vi "Three part.vi"() -> ()   [LabVIEW 2009]
uses:
  <vilib>/vision/Image Controls.llb/IMAQ Image.ctl
  <vilib>/Instr/_visa.llb/VISA Configure Serial Port (Instr).vi
  <vilib>/Analysis/3filter.llb/Filter Passband Type.ctl
  <vilib>/Analysis/3filter.llb/Butterworth Filter (DBL).vi
  <vilib>/vision/NI_Vision_Development_Module.lvlib
  <vilib>/Analysis/NI_AALBase.lvlib
panel:
  in  "Orange Guitar":T1={"Global Rectangle"=[587, 282, 628, 378], "Contours"=[{"ID"=enum."External", "Type"=2, "Coordinates"=[627, 377, 587, 282]}]} {"Contours"."Type" items=["No Selection", "Point", "Line", "Rectangle", "Oval", "Polygon", "Freehand Region", "Annulus", "Unused2", "Unused3", "Broken Line", "Freehand Line", "Rotated Rectangle"]}
  in  "Yellow Guitar":T1={"Global Rectangle"=[546, 282, 563, 376], "Contours"=[{"ID"=enum."External", "Type"=2, "Coordinates"=[562, 375, 546, 282]}]} {"Contours"."Type" items=["No Selection", "Point", "Line", "Rectangle", "Oval", "Polygon", "Freehand Region", "Annulus", "Unused2", "Unused3", "Broken Line", "Freehand Line", "Rotated Rectangle"]}
  in  "Green Guitar":T1={"Global Rectangle"=[498, 284, 505, 376], "Contours"=[{"ID"=enum."External", "Type"=2, "Coordinates"=[498, 375, 504, 284]}]} {"Contours"."Type" items=["No Selection", "Point", "Line", "Rectangle", "Oval", "Polygon", "Freehand Region", "Annulus", "Unused2", "Unused3", "Broken Line", "Freehand Line", "Rotated Rectangle"]}
  in  "Blue Guitar":T1={"Global Rectangle"=[569, 290, 594, 372], "Contours"=[{"ID"=enum."External", "Type"=2, "Coordinates"=[593, 371, 569, 290]}]} {"Contours"."Type" items=["No Selection", "Point", "Line", "Rectangle", "Oval", "Polygon", "Freehand Region", "Annulus", "Unused2", "Unused3", "Broken Line", "Freehand Line", "Rotated Rectangle"]}
  in  "Red Guitar":T1={"Global Rectangle"=[526, 284, 530, 370], "Contours"=[{"ID"=enum."External", "Type"=2, "Coordinates"=[529, 369, 526, 284]}]} {"Contours"."Type" items=["No Selection", "Point", "Line", "Rectangle", "Oval", "Polygon", "Freehand Region", "Annulus", "Unused2", "Unused3", "Broken Line", "Freehand Line", "Rotated Rectangle"]}
  in  "sampling  9":dbl=1.0 format="%0.2f"
  in  "high 14":dbl=60.0 format="%0.2f"
  out "Blue Guitar":dbl[](graph)
  in  "low 3":dbl=0.12500000000000006 format="%0.4f"
  out "Yellow Guitar":dbl[](graph)
  out "Yellow Guitar LED":bool
  in  "sampling 12":dbl=1.0 format="%0.2f"
  in  "high 13":dbl=60.0 format="%0.2f"
  in  "low  12":dbl=0.12500000000000006 format="%0.4f"
  out "Yellow Guitar":T1={"Global Rectangle"=[243, 262, 261, 384], "Contours"=[{"ID"=enum."External", "Type"=2, "Coordinates"=[260, 383, 243, 262]}]} {"Contours"."Type" items=["No Selection", "Point", "Line", "Rectangle", "Oval", "Polygon", "Freehand Region", "Annulus", "Unused2", "Unused3", "Broken Line", "Freehand Line", "Rotated Rectangle"]}
  out "Blue Guitar":T1={"Global Rectangle"=[168, 264, 180, 378], "Contours"=[{"ID"=enum."External", "Type"=2, "Coordinates"=[168, 377, 179, 264]}]} {"Contours"."Type" items=["No Selection", "Point", "Line", "Rectangle", "Oval", "Polygon", "Freehand Region", "Annulus", "Unused2", "Unused3", "Broken Line", "Freehand Line", "Rotated Rectangle"]}
  out "Green Guitar":dbl[](graph)
  out "Green Guitar LED":bool
  in  "sampling 11":dbl=1.0 format="%0.2f"
  in  "high 12":dbl=60.0 format="%0.2f"
  in  "low  11":dbl=0.12500000000000006 format="%0.4f"
  out "Green Guitar":T1={"Global Rectangle"=[406, 309, 423, 383], "Contours"=[{"ID"=enum."External", "Type"=2, "Coordinates"=[422, 382, 406, 309]}]} {"Contours"."Type" items=["No Selection", "Point", "Line", "Rectangle", "Oval", "Polygon", "Freehand Region", "Annulus", "Unused2", "Unused3", "Broken Line", "Freehand Line", "Rotated Rectangle"]}
  out "Red Guitar":dbl[](graph)
  out "Red Guitar LED":bool
  in  "sampling 10":dbl=1.0 format="%0.2f"
  in  "high 11":dbl=60.0 format="%0.2f"
  in  "low  10":dbl=0.12500000000000006 format="%0.4f"
  out "Red Guitar":T1={"Global Rectangle"=[300, 297, 320, 380], "Contours"=[{"ID"=enum."External", "Type"=2, "Coordinates"=[300, 379, 319, 297]}]} {"Contours"."Type" items=["No Selection", "Point", "Line", "Rectangle", "Oval", "Polygon", "Freehand Region", "Annulus", "Unused2", "Unused3", "Broken Line", "Freehand Line", "Rotated Rectangle"]}
  out "Blue Guitar LED":bool
  out "Orange Guitar":dbl[](graph)
  out "Orange Guitar LED":bool
  in  "sampling 9":dbl=1.0 format="%0.2f"
  in  "high 10":dbl=60.0 format="%0.2f"
  in  "low  9":dbl=0.12500000000000006 format="%0.4f"
  out "Orange Guitar":T1={"Global Rectangle"=[300, 297, 320, 380], "Contours"=[{"ID"=enum."External", "Type"=2, "Coordinates"=[300, 379, 319, 297]}]} {"Contours"."Type" items=["No Selection", "Point", "Line", "Rectangle", "Oval", "Polygon", "Freehand Region", "Annulus", "Unused2", "Unused3", "Broken Line", "Freehand Line", "Rotated Rectangle"]}
  in  "Orange Bass":T1={"Global Rectangle"=[220, 296, 225, 371], "Contours"=[{"ID"=enum."External", "Type"=2, "Coordinates"=[224, 370, 220, 296]}]} {"Contours"."Type" items=["No Selection", "Point", "Line", "Rectangle", "Oval", "Polygon", "Freehand Region", "Annulus", "Unused2", "Unused3", "Broken Line", "Freehand Line", "Rotated Rectangle"]}
  out "Orange Bass":dbl[](graph)
  out "Orange Bass LED":bool
  in  "sampling 8":dbl=1.0 format="%0.2f"
  in  "high 9":dbl=60.0 format="%0.2f"
  in  "low  8":dbl=0.12500000000000006 format="%0.4f"
  out "Orange Bass":T1={"Global Rectangle"=[300, 297, 320, 380], "Contours"=[{"ID"=enum."External", "Type"=2, "Coordinates"=[300, 379, 319, 297]}]} {"Contours"."Type" items=["No Selection", "Point", "Line", "Rectangle", "Oval", "Polygon", "Freehand Region", "Annulus", "Unused2", "Unused3", "Broken Line", "Freehand Line", "Rotated Rectangle"]}
  in  "Green Bass":T1={"Global Rectangle"=[100, 292, 131, 371], "Contours"=[{"ID"=enum."External", "Type"=2, "Coordinates"=[100, 370, 130, 292]}]} {"Contours"."Type" items=["No Selection", "Point", "Line", "Rectangle", "Oval", "Polygon", "Freehand Region", "Annulus", "Unused2", "Unused3", "Broken Line", "Freehand Line", "Rotated Rectangle"]}
  in  "Blue Bass":T1={"Global Rectangle"=[193, 293, 199, 374], "Contours"=[{"ID"=enum."External", "Type"=2, "Coordinates"=[193, 373, 198, 293]}]} {"Contours"."Type" items=["No Selection", "Point", "Line", "Rectangle", "Oval", "Polygon", "Freehand Region", "Annulus", "Unused2", "Unused3", "Broken Line", "Freehand Line", "Rotated Rectangle"]}
  in  "Red Bass":T1={"Global Rectangle"=[129, 294, 154, 376], "Contours"=[{"ID"=enum."External", "Type"=2, "Coordinates"=[129, 375, 153, 294]}]} {"Contours"."Type" items=["No Selection", "Point", "Line", "Rectangle", "Oval", "Polygon", "Freehand Region", "Annulus", "Unused2", "Unused3", "Broken Line", "Freehand Line", "Rotated Rectangle"]}
  in  "Yellow Bass":T1={"Global Rectangle"=[160, 295, 175, 378], "Contours"=[{"ID"=enum."External", "Type"=2, "Coordinates"=[160, 377, 174, 295]}]} {"Contours"."Type" items=["No Selection", "Point", "Line", "Rectangle", "Oval", "Polygon", "Freehand Region", "Annulus", "Unused2", "Unused3", "Broken Line", "Freehand Line", "Rotated Rectangle"]}
  in  "sampling  8":dbl=1.0 format="%0.2f"
  in  "high 8":dbl=60.0 format="%0.2f"
  out "Blue Bass":dbl[](graph)
  in  "low 2":dbl=0.12500000000000006 format="%0.4f"
  out "Yellow Bass":dbl[](graph)
  out "Yellow Bass LED":bool
  in  "sampling 7":dbl=1.0 format="%0.2f"
  in  "high 7":dbl=60.0 format="%0.2f"
  in  "low  7":dbl=0.12500000000000006 format="%0.4f"
  out "Yellow Bass":T1={"Global Rectangle"=[243, 262, 261, 384], "Contours"=[{"ID"=enum."External", "Type"=2, "Coordinates"=[260, 383, 243, 262]}]} {"Contours"."Type" items=["No Selection", "Point", "Line", "Rectangle", "Oval", "Polygon", "Freehand Region", "Annulus", "Unused2", "Unused3", "Broken Line", "Freehand Line", "Rotated Rectangle"]}
  out "Blue Bass":T1={"Global Rectangle"=[168, 264, 180, 378], "Contours"=[{"ID"=enum."External", "Type"=2, "Coordinates"=[168, 377, 179, 264]}]} {"Contours"."Type" items=["No Selection", "Point", "Line", "Rectangle", "Oval", "Polygon", "Freehand Region", "Annulus", "Unused2", "Unused3", "Broken Line", "Freehand Line", "Rotated Rectangle"]}
  out "Green Bass":dbl[](graph)
  out "Green Bass LED":bool
  in  "sampling 6":dbl=1.0 format="%0.2f"
  in  "high 6":dbl=60.0 format="%0.2f"
  in  "low  6":dbl=0.12500000000000006 format="%0.4f"
  out "Green Bass":T1={"Global Rectangle"=[406, 309, 423, 383], "Contours"=[{"ID"=enum."External", "Type"=2, "Coordinates"=[422, 382, 406, 309]}]} {"Contours"."Type" items=["No Selection", "Point", "Line", "Rectangle", "Oval", "Polygon", "Freehand Region", "Annulus", "Unused2", "Unused3", "Broken Line", "Freehand Line", "Rotated Rectangle"]}
  out "Red Bass":dbl[](graph)
  out "Red Bass LED":bool
  in  "sampling 5":dbl=1.0 format="%0.2f"
  in  "high 5":dbl=60.0 format="%0.2f"
  in  "low  5":dbl=0.12500000000000006 format="%0.4f"
  out "Red Bass":T1={"Global Rectangle"=[300, 297, 320, 380], "Contours"=[{"ID"=enum."External", "Type"=2, "Coordinates"=[300, 379, 319, 297]}]} {"Contours"."Type" items=["No Selection", "Point", "Line", "Rectangle", "Oval", "Polygon", "Freehand Region", "Annulus", "Unused2", "Unused3", "Broken Line", "Freehand Line", "Rotated Rectangle"]}
  out "Blue Bass LED":bool
  in  "Mask":T1 {"Contours"."Type" items=["No Selection", "Point", "Line", "Rectangle", "Oval", "Polygon", "Freehand Region", "Annulus", "Unused2", "Unused3", "Broken Line", "Freehand Line", "Rotated Rectangle"]}
  out "Image 2":T2(plugin-control)
  out "Red Line":T1={"Global Rectangle"=[300, 297, 320, 380], "Contours"=[{"ID"=enum."External", "Type"=2, "Coordinates"=[300, 379, 319, 297]}]} {"Contours"."Type" items=["No Selection", "Point", "Line", "Rectangle", "Oval", "Polygon", "Freehand Region", "Annulus", "Unused2", "Unused3", "Broken Line", "Freehand Line", "Rotated Rectangle"]}
  in  "Red Line":T1={"Global Rectangle"=[300, 297, 320, 380], "Contours"=[{"ID"=enum."External", "Type"=2, "Coordinates"=[300, 379, 319, 297]}]} {"Contours"."Type" items=["No Selection", "Point", "Line", "Rectangle", "Oval", "Polygon", "Freehand Region", "Annulus", "Unused2", "Unused3", "Broken Line", "Freehand Line", "Rotated Rectangle"]}
  out "Waveform Red":dbl[](graph)
  out "LED Red":bool
  in  "sampling 4":dbl=1.0 format="%0.2f"
  in  "high 4":dbl=60.0 format="%0.2f"
  in  "low  4":dbl=0.12500000000000006 format="%0.4f"
  out "Green Line":T1={"Global Rectangle"=[406, 309, 423, 383], "Contours"=[{"ID"=enum."External", "Type"=2, "Coordinates"=[422, 382, 406, 309]}]} {"Contours"."Type" items=["No Selection", "Point", "Line", "Rectangle", "Oval", "Polygon", "Freehand Region", "Annulus", "Unused2", "Unused3", "Broken Line", "Freehand Line", "Rotated Rectangle"]}
  in  "Blue Line":T1={"Global Rectangle"=[374, 278, 383, 377], "Contours"=[{"ID"=enum."External", "Type"=2, "Coordinates"=[382, 376, 374, 278]}]} {"Contours"."Type" items=["No Selection", "Point", "Line", "Rectangle", "Oval", "Polygon", "Freehand Region", "Annulus", "Unused2", "Unused3", "Broken Line", "Freehand Line", "Rotated Rectangle"]}
  in  "Green Line":T1={"Global Rectangle"=[406, 309, 423, 383], "Contours"=[{"ID"=enum."External", "Type"=2, "Coordinates"=[422, 382, 406, 309]}]} {"Contours"."Type" items=["No Selection", "Point", "Line", "Rectangle", "Oval", "Polygon", "Freehand Region", "Annulus", "Unused2", "Unused3", "Broken Line", "Freehand Line", "Rotated Rectangle"]}
  in  "low  3":dbl=0.12500000000000006 format="%0.4f"
  out "Waveform Green":dbl[](graph)
  out "LED Green":bool
  in  "sampling 3":dbl=1.0 format="%0.2f"
  in  "high 3":dbl=60.0 format="%0.2f"
  in  "Yellow Line":T1={"Global Rectangle"=[342, 292, 349, 377], "Contours"=[{"ID"=enum."External", "Type"=2, "Coordinates"=[342, 376, 348, 292]}]} {"Contours"."Type" items=["No Selection", "Point", "Line", "Rectangle", "Oval", "Polygon", "Freehand Region", "Annulus", "Unused2", "Unused3", "Broken Line", "Freehand Line", "Rotated Rectangle"]}
  out "Blue Line":T1={"Global Rectangle"=[168, 264, 180, 378], "Contours"=[{"ID"=enum."External", "Type"=2, "Coordinates"=[168, 377, 179, 264]}]} {"Contours"."Type" items=["No Selection", "Point", "Line", "Rectangle", "Oval", "Polygon", "Freehand Region", "Annulus", "Unused2", "Unused3", "Broken Line", "Freehand Line", "Rotated Rectangle"]}
  out "cluster":T3
  in  "baud rate (9600)":u32=9600
  in  "VISA resource name":refnum<visa-resource-name>
  out "number":u32
  out "decimal integer string":string
  out "Image Dst Out":T2
  out "Yellow Line":T1={"Global Rectangle"=[243, 262, 261, 384], "Contours"=[{"ID"=enum."External", "Type"=2, "Coordinates"=[260, 383, 243, 262]}]} {"Contours"."Type" items=["No Selection", "Point", "Line", "Rectangle", "Oval", "Polygon", "Freehand Region", "Annulus", "Unused2", "Unused3", "Broken Line", "Freehand Line", "Rotated Rectangle"]}
  in  "low  2":dbl=0.12500000000000006 format="%0.4f"
  in  "high 2":dbl=60.0 format="%0.2f"
  in  "sampling 2":dbl=1.0 format="%0.2f"
  out "LED Yellow":bool
  out "Waveform Yellow":dbl[](graph)
  in  "playtime":dbl=30.0
  out "Frame Number":i32
  in  "Frame Start":i32=2400
  out "Blue Drum":bool
  in  "low":dbl=0.12500000000000006 format="%0.4f"
  out "Blue Drum":dbl[](graph)
  in  "high":dbl=60.0 format="%0.2f"
  in  "sampling":dbl=1.0 format="%0.2f"
  in  "stop":bool
  in  "AVI Path":path
  # "BLUE"
  # "YELLOW"
  # "GREEN"
  # "RED"
  # "Drums"
  # "Bass"
  # "Guitar"
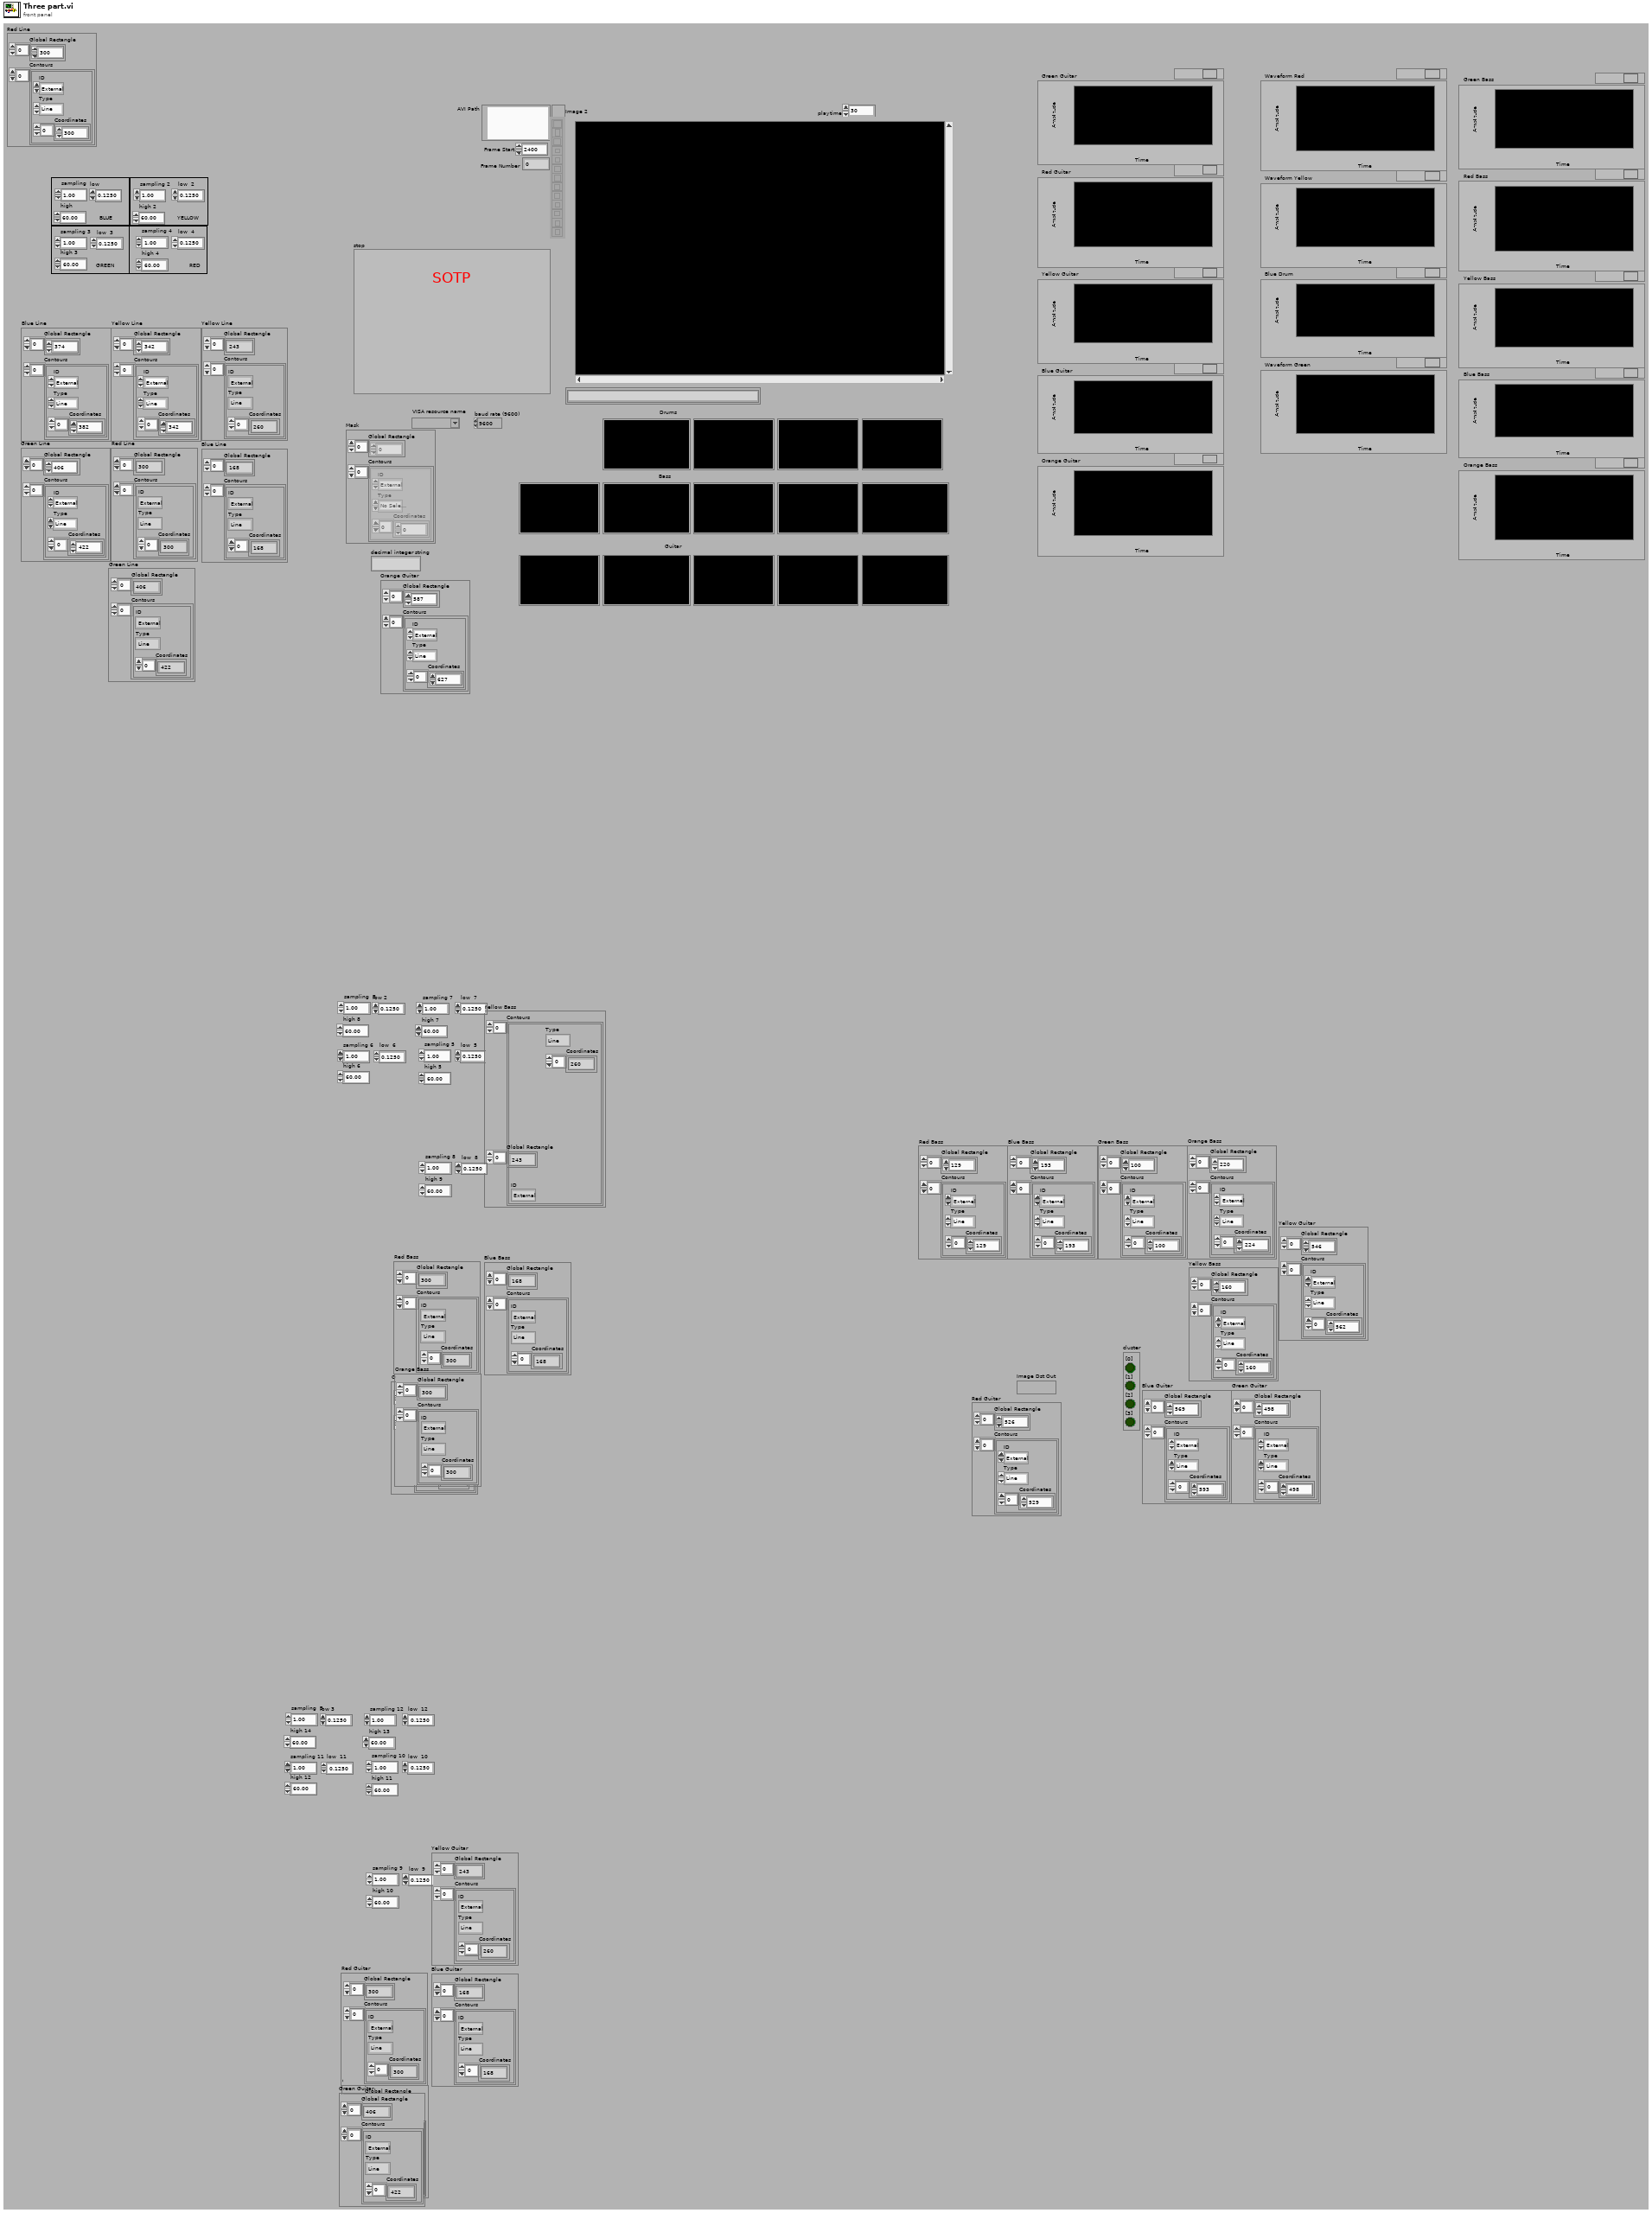
[diagram p1: front panel]
types:
  T1 = cluster{"Global Rectangle":i32[], "Contours":cluster{"ID":enum32{"External", "Internal"}, "Type":u32, "Coordinates":i32[]}[]}
  T2 = typedef "IMAQ Image.ctl" = refnum<image>
  T3 = cluster{"[0]":bool, "[1]":bool, "[2]":bool, "[3]":bool, "[4]":bool, "[5]":bool, "[6]":bool, "[7]":bool, "[8]":bool}
  T4 = typedef "NI_AALBase.lvlib/Filter Passband Type.ctl" = enum32{"Lowpass", "Highpass", "Bandpass", "Bandstop"}
  T5 = cluster{"Left":i32, "Top":i32, "Right":i32, "Bottom":i32}
  T6 = typedef "Image Type" = u32
  T7 = typedef "AviRefnum.ctl" = refnum<k1>
  T8 = cluster{"ID":enum32{"External", "Internal"}, "Type":u32, "Coordinates":i32[]}[]
  T9 = cluster{"ID":enum32{"External", "Internal"}, "Type":u32, "Coordinates":i32[]}
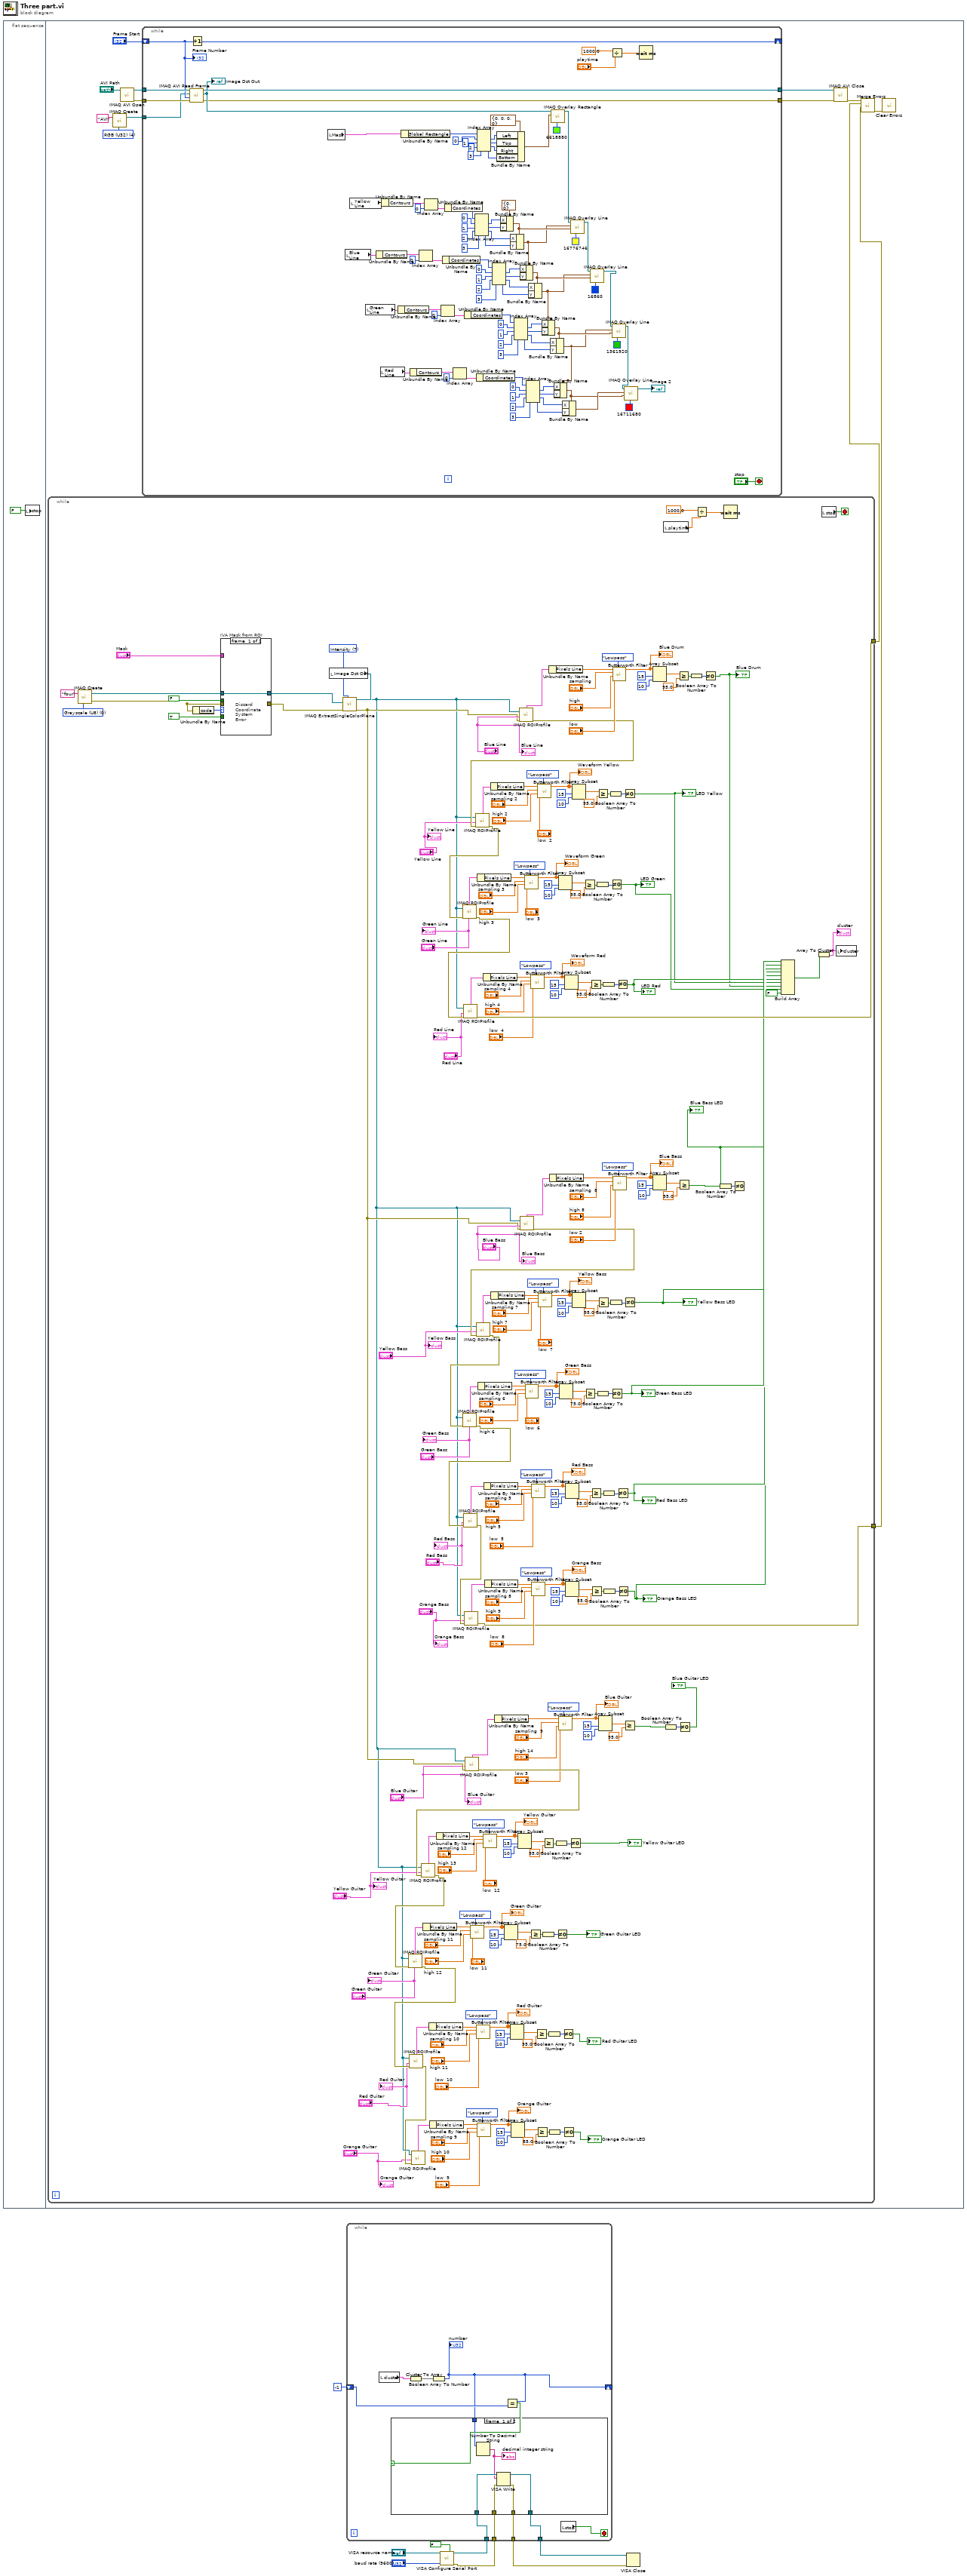
[diagram p0: block diagram]
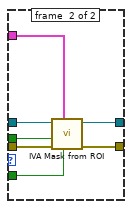
[diagram p3: hidden frame]
diagram:
  n1 = flat-sequence {
    frame #0 {
      n2 = local write "stop"(FALSE ("stop")) -> ()
    }
    frame #1 {
      w14 = T6 4 items=["Grayscale (U8)", "Grayscale (I16)", "Grayscale (SGL)", "Complex (CSG)", "RGB (U32)", "HSL (U32)", "RGB (U64)", "Grayscale (U16)"] ("Image Type")
      n3 = while {
        tunnel: [w250] -> w11
        tunnel: [w116] -> w10
        stop <- w265 stop-if-true
        w260 = T6 0 items=["Grayscale (U8)", "Grayscale (I16)", "Grayscale (SGL)", "Complex (CSG)", "RGB (U32)", "HSL (U32)", "RGB (U64)", "Grayscale (U16)"] ("Image Type")
        w266 = 7 items=["Red", "Green", "Blue", "Hue", "Saturation", "Luminance", "Value", "Intensity"] ("Color Plane")
        n4 = call "IMAQ Create"("Image Name"="four", "Image Type"=w260) -> ("New Image"=w253:T2, "error out"=w254:errorcluster)  [unwired: 3 in]
        n5 = Unbundle By Name(w254) -> ("code"=w258:i32)
        n6 = case "IVA Mask from ROI" shown="Default" w258 {
          tunnel: "Mask" -> [_ w274]
          tunnel: TRUE ("Shrink") -> [_ w273]
          tunnel: w253 -> [w267 w272]
          tunnel: w254 -> [_ w271]
          tunnel: [_ w270] -> w255
          tunnel: [w267 w269] -> w251
          tunnel: FALSE ("Out / In") -> [_ w268]
          frame #0 {
            # "Discard\nCoordinate\nSystem\nError"
          }
          frame #1 {
            n7 = call <vilib>:"IVA Mask from ROI.vi"("Shrink"=w273, "ROI Descriptor"=w274, "error in (no error)"=w271, "Out / In"=w268, "Image Src"=w272) -> ("error out"=w270:errorcluster, "Image Out"=w269:T2)  [unwired: 5 out]
          }
        }
        n8 = local read "Image Dst Out"() -> (w261:T2)
        n9 = call "IMAQ ExtractSingleColorPlane"("Color Plane"=w266, "error in (no error)"=w255, "Image Dst"=w251, "Image Src"=w261) -> ("error out"=w31:errorcluster, "Image Dst Out"=w26:T2)  [unwired: 6 out]
        n10 = call "IMAQ ROIProfile"("error in (no error)"=w31, "ROI Descriptor"="Blue Guitar", "Image"=w26) -> ("error out"=w56:errorcluster, "ROI Graph"=w57:cluster{"x0":sgl, "dx":sgl, "Pixels Line":sgl[]})  [unwired: 4 out]
        n11 = call "IMAQ ROIProfile"("error in (no error)"=w56, "ROI Descriptor"="Yellow Guitar", "Image"=w26) -> ("error out"=w86:errorcluster, "ROI Graph"=w53:cluster{"x0":sgl, "dx":sgl, "Pixels Line":sgl[]})  [unwired: 4 out]
        n12 = call "IMAQ ROIProfile"("error in (no error)"=w86, "ROI Descriptor"="Green Guitar", "Image"=w26) -> ("error out"=w85:errorcluster, "ROI Graph"=w59:cluster{"x0":sgl, "dx":sgl, "Pixels Line":sgl[]})  [unwired: 4 out]
        n13 = call "IMAQ ROIProfile"("error in (no error)"=w85, "ROI Descriptor"="Red Guitar", "Image"=w26) -> ("error out"=w25:errorcluster, "ROI Graph"=w83:cluster{"x0":sgl, "dx":sgl, "Pixels Line":sgl[]})  [unwired: 4 out]
        n14 = call "IMAQ ROIProfile"("error in (no error)"=w25, "ROI Descriptor"="Orange Guitar", "Image"=w26) -> ("ROI Graph"=w24:cluster{"x0":sgl, "dx":sgl, "Pixels Line":sgl[]})  [unwired: 5 out]
        n15 = Unbundle By Name(w59) -> ("Pixels Line"=w62:sgl[])
        n16 = Unbundle By Name(w83) -> ("Pixels Line"=w80:sgl[])
        n17 = Unbundle By Name(w24) -> ("Pixels Line"=w90:sgl[])
        n18 = Unbundle By Name(w53) -> ("Pixels Line"=w50:sgl[])
        n19 = call-poly <vilib>:"Butterworth Filter.vi"("filter type"=Filter_Passband_Type."Lowpass", "low cutoff freq: fl"="low  11", "high cutoff freq: fh"="high 12", "sampling freq: fs"="sampling 11", "X"=w62) -> ("Filtered X"=w58:dbl[])  [unwired: 3 in, 1 out]
        "Green Guitar" <- w58
        n20 = call-poly <vilib>:"Butterworth Filter.vi"("filter type"=Filter_Passband_Type."Lowpass", "low cutoff freq: fl"="low  10", "high cutoff freq: fh"="high 11", "sampling freq: fs"="sampling 10", "X"=w80) -> ("Filtered X"=w84:dbl[])  [unwired: 3 in, 1 out]
        "Red Guitar" <- w84
        n21 = call-poly <vilib>:"Butterworth Filter.vi"("filter type"=Filter_Passband_Type."Lowpass", "low cutoff freq: fl"="low  9", "high cutoff freq: fh"="high 10", "sampling freq: fs"="sampling 9", "X"=w90) -> ("Filtered X"=w87:dbl[])  [unwired: 3 in, 1 out]
        "Orange Guitar" <- w87
        n22 = call-poly <vilib>:"Butterworth Filter.vi"("filter type"=Filter_Passband_Type."Lowpass", "low cutoff freq: fl"="low  12", "high cutoff freq: fh"="high 13", "sampling freq: fs"="sampling 12", "X"=w50) -> ("Filtered X"=w54:dbl[])  [unwired: 3 in, 1 out]
        "Yellow Guitar" <- w54
        n23 = Unbundle By Name(w57) -> ("Pixels Line"=w34:sgl[])
        n24 = Array Subset(array=w58, index=15, length=10) -> (w67:dbl[])
        n25 = Array Subset(array=w84, index=15, length=10) -> (w75:dbl[])
        n26 = Array Subset(array=w87, index=15, length=10) -> (w95:dbl[])
        n27 = Array Subset(array=w54, index=15, length=10) -> (w45:dbl[])
        n28 = call "IMAQ ROIProfile"("error in (no error)"=w31, "ROI Descriptor"="Blue Line", "Image"=w26) -> ("error out"=w225:errorcluster, "ROI Graph"=w224:cluster{"x0":sgl, "dx":sgl, "Pixels Line":sgl[]})  [unwired: 4 out]
        n29 = call "IMAQ ROIProfile"("error in (no error)"=w225, "ROI Descriptor"="Yellow Line", "Image"=w26) -> ("error out"=w192:errorcluster, "ROI Graph"=w228:cluster{"x0":sgl, "dx":sgl, "Pixels Line":sgl[]})  [unwired: 4 out]
        n30 = call "IMAQ ROIProfile"("error in (no error)"=w192, "ROI Descriptor"="Green Line", "Image"=w26) -> ("error out"=w195:errorcluster, "ROI Graph"=w222:cluster{"x0":sgl, "dx":sgl, "Pixels Line":sgl[]})  [unwired: 4 out]
        n31 = call "IMAQ ROIProfile"("error in (no error)"=w195, "ROI Descriptor"="Red Line", "Image"=w26) -> ("error out"=w250:errorcluster, "ROI Graph"=w197:cluster{"x0":sgl, "dx":sgl, "Pixels Line":sgl[]})  [unwired: 4 out]
        n32 = Unbundle By Name(w222) -> ("Pixels Line"=w219:sgl[])
        n33 = Unbundle By Name(w197) -> ("Pixels Line"=w200:sgl[])
        n34 = Unbundle By Name(w228) -> ("Pixels Line"=w231:sgl[])
        n35 = call "IMAQ ROIProfile"("error in (no error)"=w31, "ROI Descriptor"="Blue Bass", "Image"=w26) -> ("error out"=w165:errorcluster, "ROI Graph"=w164:cluster{"x0":sgl, "dx":sgl, "Pixels Line":sgl[]})  [unwired: 4 out]
        n36 = call "IMAQ ROIProfile"("error in (no error)"=w165, "ROI Descriptor"="Yellow Bass", "Image"=w26) -> ("error out"=w135:errorcluster, "ROI Graph"=w168:cluster{"x0":sgl, "dx":sgl, "Pixels Line":sgl[]})  [unwired: 4 out]
        n37 = call "IMAQ ROIProfile"("error in (no error)"=w135, "ROI Descriptor"="Green Bass", "Image"=w26) -> ("error out"=w136:errorcluster, "ROI Graph"=w162:cluster{"x0":sgl, "dx":sgl, "Pixels Line":sgl[]})  [unwired: 4 out]
        n38 = call "IMAQ ROIProfile"("error in (no error)"=w136, "ROI Descriptor"="Red Bass", "Image"=w26) -> ("error out"=w117:errorcluster, "ROI Graph"=w138:cluster{"x0":sgl, "dx":sgl, "Pixels Line":sgl[]})  [unwired: 4 out]
        n39 = call "IMAQ ROIProfile"("error in (no error)"=w117, "ROI Descriptor"="Orange Bass", "Image"=w26) -> ("error out"=w116:errorcluster, "ROI Graph"=w129:cluster{"x0":sgl, "dx":sgl, "Pixels Line":sgl[]})  [unwired: 4 out]
        n40 = Unbundle By Name(w162) -> ("Pixels Line"=w159:sgl[])
        n41 = Unbundle By Name(w138) -> ("Pixels Line"=w141:sgl[])
        n42 = Unbundle By Name(w129) -> ("Pixels Line"=w126:sgl[])
        n43 = Unbundle By Name(w168) -> ("Pixels Line"=w171:sgl[])
        n44 = call-poly <vilib>:"Butterworth Filter.vi"("filter type"=Filter_Passband_Type."Lowpass", "low cutoff freq: fl"="low  3", "high cutoff freq: fh"="high 3", "sampling freq: fs"="sampling 3", "X"=w219) -> ("Filtered X"=w223:dbl[])  [unwired: 3 in, 1 out]
        "Waveform Green" <- w223
        n45 = call-poly <vilib>:"Butterworth Filter.vi"("filter type"=Filter_Passband_Type."Lowpass", "low cutoff freq: fl"="low  6", "high cutoff freq: fh"="high 6", "sampling freq: fs"="sampling 6", "X"=w159) -> ("Filtered X"=w163:dbl[])  [unwired: 3 in, 1 out]
        "Green Bass" <- w163
        n46 = Greater Or Equal?(x=w67, y=75.0) -> (x >= y?=w65:bool[])
        n47 = call-poly <vilib>:"Butterworth Filter.vi"("filter type"=Filter_Passband_Type."Lowpass", "low cutoff freq: fl"="low  4", "high cutoff freq: fh"="high 4", "sampling freq: fs"="sampling 4", "X"=w200) -> ("Filtered X"=w196:dbl[])  [unwired: 3 in, 1 out]
        "Waveform Red" <- w196
        n48 = call-poly <vilib>:"Butterworth Filter.vi"("filter type"=Filter_Passband_Type."Lowpass", "low cutoff freq: fl"="low  5", "high cutoff freq: fh"="high 5", "sampling freq: fs"="sampling 5", "X"=w141) -> ("Filtered X"=w137:dbl[])  [unwired: 3 in, 1 out]
        "Red Bass" <- w137
        n49 = call-poly <vilib>:"Butterworth Filter.vi"("filter type"=Filter_Passband_Type."Lowpass", "low cutoff freq: fl"="low  8", "high cutoff freq: fh"="high 9", "sampling freq: fs"="sampling 8", "X"=w126) -> ("Filtered X"=w130:dbl[])  [unwired: 3 in, 1 out]
        "Orange Bass" <- w130
        n50 = Greater Or Equal?(x=w75, y=95.0) -> (x >= y?=w77:bool[])
        n51 = Greater Or Equal?(x=w95, y=85.0) -> (x >= y?=w93:bool[])
        n52 = call-poly <vilib>:"Butterworth Filter.vi"("filter type"=Filter_Passband_Type."Lowpass", "low cutoff freq: fl"="low  2", "high cutoff freq: fh"="high 2", "sampling freq: fs"="sampling 2", "X"=w231) -> ("Filtered X"=w227:dbl[])  [unwired: 3 in, 1 out]
        "Waveform Yellow" <- w227
        n53 = call-poly <vilib>:"Butterworth Filter.vi"("filter type"=Filter_Passband_Type."Lowpass", "low cutoff freq: fl"="low  7", "high cutoff freq: fh"="high 7", "sampling freq: fs"="sampling 7", "X"=w171) -> ("Filtered X"=w167:dbl[])  [unwired: 3 in, 1 out]
        "Yellow Bass" <- w167
        n54 = Boolean Array To Number(Boolean array=w65) -> (number=w64:u32)
        n55 = Greater Or Equal?(x=w45, y=95.0) -> (x >= y?=w47:bool[])
        n56 = Boolean Array To Number(Boolean array=w77) -> (number=w78:u32)
        n57 = Boolean Array To Number(Boolean array=w93) -> (number=w92:u32)
        n58 = Unbundle By Name(w224) -> ("Pixels Line"=w248:sgl[])
        n59 = Unbundle By Name(w164) -> ("Pixels Line"=w187:sgl[])
        n60 = Boolean Array To Number(Boolean array=w47) -> (number=w48:u32)
        n61 = Not Equal To 0?(x=w64) -> (x != 0?=→"Green Guitar LED":bool)
        n62 = call-poly <vilib>:"Butterworth Filter.vi"("filter type"=Filter_Passband_Type."Lowpass", "low cutoff freq: fl"="low 3", "high cutoff freq: fh"="high 14", "sampling freq: fs"="sampling  9", "X"=w34) -> ("Filtered X"=w71:dbl[])  [unwired: 3 in, 1 out]
        "Blue Guitar" <- w71
        n63 = Array Subset(array=w223, index=15, length=10) -> (w214:dbl[])
        n64 = Array Subset(array=w163, index=15, length=10) -> (w154:dbl[])
        n65 = Not Equal To 0?(x=w78) -> (x != 0?=→"Red Guitar LED":bool)
        n66 = Not Equal To 0?(x=w92) -> (x != 0?=→"Orange Guitar LED":bool)
        n67 = Array Subset(array=w196, index=15, length=10) -> (w205:dbl[])
        n68 = Array Subset(array=w137, index=15, length=10) -> (w146:dbl[])
        n69 = Array Subset(array=w130, index=15, length=10) -> (w121:dbl[])
        n70 = Not Equal To 0?(x=w48) -> (x != 0?=→"Yellow Guitar LED":bool)
        n71 = Array Subset(array=w227, index=15, length=10) -> (w236:dbl[])
        n72 = Array Subset(array=w167, index=15, length=10) -> (w176:dbl[])
        n73 = Greater Or Equal?(x=w214, y=95.0) -> (x >= y?=w216:bool[])
        n74 = Greater Or Equal?(x=w154, y=75.0) -> (x >= y?=w156:bool[])
        n75 = Greater Or Equal?(x=w205, y=95.0) -> (x >= y?=w203:bool[])
        n76 = Greater Or Equal?(x=w146, y=95.0) -> (x >= y?=w144:bool[])
        n77 = Greater Or Equal?(x=w121, y=85.0) -> (x >= y?=w123:bool[])
        n78 = Boolean Array To Number(Boolean array=w216) -> (number=w217:u32)
        n79 = Greater Or Equal?(x=w236, y=95.0) -> (x >= y?=w234:bool[])
        n80 = Boolean Array To Number(Boolean array=w156) -> (number=w157:u32)
        n81 = Greater Or Equal?(x=w176, y=95.0) -> (x >= y?=w174:bool[])
        n82 = Array Subset(array=w71, index=15, length=10) -> (w40:dbl[])
        n83 = Boolean Array To Number(Boolean array=w203) -> (number=w202:u32)
        n84 = Boolean Array To Number(Boolean array=w144) -> (number=w143:u32)
        n85 = Boolean Array To Number(Boolean array=w123) -> (number=w124:u32)
        n86 = Boolean Array To Number(Boolean array=w234) -> (number=w233:u32)
        n87 = Boolean Array To Number(Boolean array=w174) -> (number=w173:u32)
        n88 = Not Equal To 0?(x=w217) -> (x != 0?=w106:bool)
        "LED Green" <- w106
        n89 = Not Equal To 0?(x=w157) -> (x != 0?=w114:bool)
        "Green Bass LED" <- w114
        n90 = call-poly <vilib>:"Butterworth Filter.vi"("filter type"=Filter_Passband_Type."Lowpass", "low cutoff freq: fl"="low", "high cutoff freq: fh"="high", "sampling freq: fs"="sampling", "X"=w248) -> ("Filtered X"=w210:dbl[])  [unwired: 3 in, 1 out]
        "Blue Drum" <- w210
        n91 = call-poly <vilib>:"Butterworth Filter.vi"("filter type"=Filter_Passband_Type."Lowpass", "low cutoff freq: fl"="low 2", "high cutoff freq: fh"="high 8", "sampling freq: fs"="sampling  8", "X"=w187) -> ("Filtered X"=w150:dbl[])  [unwired: 3 in, 1 out]
        "Blue Bass" <- w150
        n92 = Not Equal To 0?(x=w202) -> (x != 0?=w109:bool)
        "LED Red" <- w109
        n93 = Not Equal To 0?(x=w143) -> (x != 0?=w113:bool)
        "Red Bass LED" <- w113
        n94 = Not Equal To 0?(x=w124) -> (x != 0?=w110:bool)
        "Orange Bass LED" <- w110
        n95 = Not Equal To 0?(x=w233) -> (x != 0?=w108:bool)
        "LED Yellow" <- w108
        n96 = Greater Or Equal?(x=w40, y=95.0) -> (x >= y?=w103:bool[])
        n97 = Not Equal To 0?(x=w173) -> (x != 0?=w112:bool)
        "Yellow Bass LED" <- w112
        n98 = Array Subset(array=w210, index=15, length=10) -> (w242:dbl[])
        n99 = Array Subset(array=w150, index=15, length=10) -> (w181:dbl[])
        n100 = local read "playtime"() -> (w262:dbl)
        n101 = Boolean Array To Number(Boolean array=w103) -> (number=w42:u32)
        n102 = Greater Or Equal?(x=w242, y=95.0) -> (x >= y?=w240:bool[])
        n103 = Greater Or Equal?(x=w181, y=95.0) -> (x >= y?=w104:bool[])
        n104 = Not Equal To 0?(x=w42) -> (x != 0?=→"Blue Guitar LED":bool)
        n105 = Boolean Array To Number(Boolean array=w240) -> (number=w239:u32)
        n106 = Divide(x=1000.0, y=w262) -> (x/y=w264:dbl)
        n107 = Not Equal To 0?(x=w239) -> (x != 0?=w107:bool)
        "Blue Drum" <- w107
        n108 = Boolean Array To Number(Boolean array=w104) -> (number=w179:u32)
        n109 = Wait (ms)(milliseconds to wait=w264) -> ()  [unwired: 1 out]
        n110 = Not Equal To 0?(x=w179) -> (x != 0?=w111:bool)
        "Blue Bass LED" <- w111
        n111 = Build Array(w114, w113, w112, w111, w110, w109, w108, w107, w106, FALSE ("element")) -> (w190:bool[])
        n112 = Array To Cluster(array=w190) -> (cluster=w191:T3)
        "cluster" <- w191
        n113 = local read "stop"() -> (w265:bool)
        n114 = local write "cluster"(w191) -> ()
        "Yellow Line" <- "Yellow Line"
        "Blue Line" <- "Blue Line"
        "Green Line" <- "Green Line"
        "Red Line" <- "Red Line"
        "Yellow Bass" <- "Yellow Bass"
        "Blue Bass" <- "Blue Bass"
        "Green Bass" <- "Green Bass"
        "Red Bass" <- "Red Bass"
        "Orange Bass" <- "Orange Bass"
        "Yellow Guitar" <- "Yellow Guitar"
        "Blue Guitar" <- "Blue Guitar"
        "Green Guitar" <- "Green Guitar"
        "Red Guitar" <- "Red Guitar"
        "Orange Guitar" <- "Orange Guitar"
      }
      n115 = call "IMAQ Create"("Image Name"="AVI", "Image Type"=w14) -> ("New Image"=w12:T2)  [unwired: 3 in, 1 out]
      n116 = call "IMAQ AVI Open"("AVI Path"="AVI Path") -> ("error out"=w19:errorcluster, "Avi Refnum"=w20:T7)  [unwired: 9 in]
      n117 = while {
        tunnel: w20 -> [w369]
        tunnel: w19 -> [w317]
        tunnel: [w368] -> w21
        shift-right: [w363] -> _
        shift-left: "Frame Start" -> [w362]
        tunnel: [w313] -> w15
        tunnel: w12 -> [w312]
        stop <- "stop" stop-if-true
        n118 = call "IMAQ AVI Read Frame"("error in (no error)"=w317, "Frame Number"=w362, "Image"=w312, "Avi Refnum"=w369) -> ("error out"=w313:errorcluster, "Image Out"=w314:T2, "Avi Refnum (duplicate)"=w368:T7)  [unwired: 4 in, 1 out]
        "Image Dst Out" <- w314
        n119 = Increment(x=w362) -> (x+1=w363:i32)
        n120 = local read "Mask"() -> (w275:T1)
        n121 = local read "Blue Line"() -> (w316:T1)
        n122 = local read "Yellow Line"() -> (w315:T1)
        n123 = local read "Green Line"() -> (w311:T1)
        n124 = Unbundle By Name(w316) -> ("Contours"=w329:T8)
        n125 = local read "Red Line"() -> (w278:T1)
        n126 = Unbundle By Name(w315) -> ("Contours"=w344:T8)
        n127 = Unbundle By Name(w311) -> ("Contours"=w301:T8)
        n128 = Unbundle By Name(w275) -> ("Global Rectangle"=w358:i32[])
        n129 = Unbundle By Name(w278) -> ("Contours"=w288:T8)
        n130 = Index Array(array=w329, index=0) -> (element=w328:T9)
        n131 = Index Array(array=w344, index=0) -> (element=w346:T9)
        n132 = Index Array(array=w301, index=0) -> (element=w302:T9)
        n133 = Unbundle By Name(w328) -> ("Coordinates"=w327:i32[])
        n134 = Unbundle By Name(w346) -> ("Coordinates"=w347:i32[])
        n135 = Index Array(array=w288, index=0) -> (element=w287:T9)
        n136 = Unbundle By Name(w302) -> ("Coordinates"=w303:i32[])
        n137 = Index Array(array=w347, index #1=0 ("index"), index #2=1 ("index"), index #3=2 ("index"), index #4=3 ("index")) -> (element #1=w339:i32, element #2=w340:i32, element #3=w341:i32, element #4=w342:i32)
        n138 = Unbundle By Name(w287) -> ("Coordinates"=w286:i32[])
        n139 = Index Array(array=w358, index #1=0 ("index"), index #2=1 ("index"), index #3=2 ("index"), index #4=3 ("index")) -> (element #1=w357:i32, element #2=w356:i32, element #3=w355:i32, element #4=w354:i32)
        n140 = Index Array(array=w327, index #1=0 ("index"), index #2=1 ("index"), index #3=2 ("index"), index #4=3 ("index")) -> (element #1=w326:i32, element #2=w332:i32, element #3=w331:i32, element #4=w330:i32)
        n141 = Bundle By Name(cluster=T5 {"Left"=0, "Top"=0, "Right"=0, "Bottom"=0} ("Rectangle"), "Left"=w357, "Top"=w356, "Right"=w355, "Bottom"=w354) -> (w360:T5)
        n142 = Bundle By Name(cluster=cluster{"X":i32, "Y":i32} {"X"=0, "Y"=0} ("End Point"), "X"=w339, "Y"=w340) -> (w348:cluster{"X":i32, "Y":i32})
        n143 = Bundle By Name(cluster=w348, "X"=w341, "Y"=w342) -> (w319:cluster{"X":i32, "Y":i32})
        n144 = Index Array(array=w303, index #1=0 ("index"), index #2=1 ("index"), index #3=2 ("index"), index #4=3 ("index")) -> (element #1=w304:i32, element #2=w298:i32, element #3=w299:i32, element #4=w300:i32)
        n145 = Bundle By Name(cluster=w319, "X"=w326, "Y"=w332) -> (w333:cluster{"X":i32, "Y":i32})
        n146 = Index Array(array=w286, index #1=0 ("index"), index #2=1 ("index"), index #3=2 ("index"), index #4=3 ("index")) -> (element #1=w285:i32, element #2=w291:i32, element #3=w290:i32, element #4=w289:i32)
        n147 = Bundle By Name(cluster=w333, "X"=w331, "Y"=w330) -> (w296:cluster{"X":i32, "Y":i32})
        n148 = Bundle By Name(cluster=w296, "X"=w304, "Y"=w298) -> (w295:cluster{"X":i32, "Y":i32})
        n149 = Bundle By Name(cluster=w295, "X"=w299, "Y"=w300) -> (w277:cluster{"X":i32, "Y":i32})
        n150 = call "IMAQ Overlay Rectangle"("Color"=u32 6618880, "Rectangle"=w360, "Image"=w314) -> ("Image Out"=w334:T2)  [unwired: 7 in, 1 out]
        n151 = Bundle By Name(cluster=w277, "X"=w285, "Y"=w291) -> (w293:cluster{"X":i32, "Y":i32})
        n152 = Bundle By Name(cluster=w293, "X"=w290, "Y"=w289) -> (w294:cluster{"X":i32, "Y":i32})
        n153 = call "IMAQ Overlay Line"("Color"=u32 16776746, "End Point"=w348, "Start Point"=w319, "Image"=w334) -> ("Image Out"=w324:T2)  [unwired: 6 in, 1 out]
        n154 = call "IMAQ Overlay Line"("Color"=u32 16860, "End Point"=w333, "Start Point"=w296, "Image"=w324) -> ("Image Out"=w297:T2)  [unwired: 6 in, 1 out]
        n155 = Divide(x=1000.0, y="playtime") -> (x/y=w366:dbl)
        n156 = call "IMAQ Overlay Line"("Color"=u32 1361920, "End Point"=w295, "Start Point"=w277, "Image"=w297) -> ("Image Out"=w276:T2)  [unwired: 6 in, 1 out]
        n157 = call "IMAQ Overlay Line"("Color"=u32 16711680, "End Point"=w293, "Start Point"=w294, "Image"=w276) -> ("Image Out"=→"Image 2":T2)  [unwired: 6 in, 1 out]
        n158 = Wait (ms)(milliseconds to wait=w366) -> ()  [unwired: 1 out]
        "Frame Number" <- w362
      }
      n159 = call "IMAQ AVI Close"("error in (no error)"=w15, "Avi Refnum"=w21) -> ("error out"=w17:errorcluster)  [unwired: 9 in]
      n160 = call <vilib>:"Merge Errors.vi"("error in 3 (no error)"=w10, "error in 2 (no error)"=w11, "error in 1 (no error)"=w17) -> ("error out"=w16:errorcluster)  [unwired: 4 in]
      n161 = call <vilib>:"Clear Errors.vi"("error in (no error)"=w16) -> ()  [unwired: 6 in, 1 out]
    }
  }
  n162 = call-poly "VISA Configure Serial Port"("VISA resource name"="VISA resource name", "Enable Termination\nChar (T)"=FALSE ("Enable Termination\nChar (T)"), "baud rate (9600)"="baud rate (9600)") -> ("VISA resource name out"=w7:refnum<visa-resource-name>, "error out"=w2:errorcluster)  [unwired: 11 in]
  n163 = while {
    shift-right: [w373] -> _
    shift-left: -1 -> [w379]
    tunnel: w7 -> [w377]
    tunnel: [w376] -> w6
    tunnel: w2 -> [w375]
    tunnel: [w374] -> w1
    stop <- w370 stop-if-true
    n164 = local read "cluster"() -> (w371:T3)
    n165 = Cluster To Array(cluster=w371) -> (array=w372:bool[])
    n166 = Boolean Array To Number(Boolean array=w372) -> (number=w373:u32)
    "number" <- w373
    n167 = Equal?(x=w373, y=w379) -> (x = y?=w378:bool)
    n168 = case shown="False" w378 {
      tunnel: w377 -> [w385 w387]
      tunnel: [w384 w387] -> w376
      tunnel: w373 -> [w382 _]
      tunnel: w375 -> [w381 w386]
      tunnel: [w380 w386] -> w374
      frame #0 {
        n169 = Number To Decimal String(number=w382) -> (decimal integer string=w383:string)  [unwired: 1 in]
        "decimal integer string" <- w383
        n170 = VISA Write(VISA resource name=w385, write buffer=w383, error in (no error)=w381) -> (VISA resource name out=w384:refnum<visa-resource-name>, error out=w380:errorcluster)  [unwired: 1 out]
      }
      frame #1 {
      }
    }
    n171 = local read "stop"() -> (w370:bool)
  }
  n172 = VISA Close(VISA resource name=w6, error in (no error)=w1) -> ()  [unwired: 1 out]
